vi "timekeeper time (g).vi"() -> ()   [LabVIEW 2011, in "EPS_Timekeeper.lvlib"]
uses:
  <vilib>/addons/Electrical Power/Example Support/PMU/Time Keeper/EPS_Timekeeper.lvlib
panel:
  out "time (ns)(g)":fxp<+,64,64>
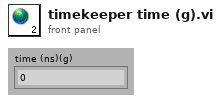
[diagram p1: front panel]
diagram:
